vi "TDMS.MoveTDMS.vi"(8 "error in (no error)":errorcluster, 10 "Target path":path, 11 "Source Path":path) -> (0 "error out":errorcluster)   [LabVIEW 2014, in "NIAnalysis.lvlib"]
uses:
  NIAnalysis.lvlib
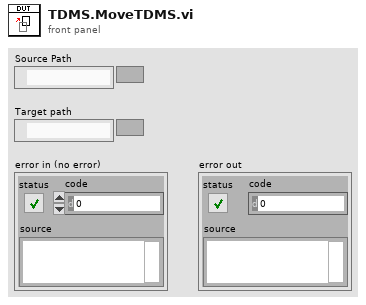
[diagram p1: front panel]
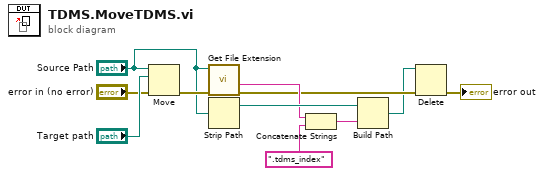
[diagram p0: block diagram]
diagram:
  n1 = Move(source path="Source Path", error in="error in (no error)", 10:"Target path") -> (error out=w10:errorcluster)  [unwired: 2 in, 2 out]
  n2 = call <vilib>:"Get File Extension.vi"("error in (no error)"=w10, "file"="Source Path") -> ("error out"=w4:errorcluster, "filename without extension"=w7:string)  [unwired: 6 in, 2 out]
  n3 = Strip Path(path="Source Path") -> (stripped path=w8:path)  [unwired: 1 out]
  n4 = Concatenate Strings(w7, ".tdms_index" ("filename without extension")) -> (w5:string)
  n5 = Build Path(base path=w8, name or relative path=w5) -> (appended path=w3:path)
  n6 = Delete(path (use dialog)=w3, error in=w4) -> (error out=→"error out":errorcluster)  [unwired: 3 in, 2 out]
